vi "FTW-WebServer-Worker-Launch.vi"(0 "Message Handler":refnum<user-event>, 5 "FTW-Endpoint in":refnum<class "FTW-Endpoint.lvclass">, 11 "error in":errorcluster) -> (15 "error out":errorcluster)   [LabVIEW 2015, in "FTW-WebServer.lvclass"]
uses:
  FTW-WebServer.lvclass
  Endpoint/FTW-Endpoint.lvclass
  Message/HttpRequest/FTW-Message-HttpRequest.lvclass
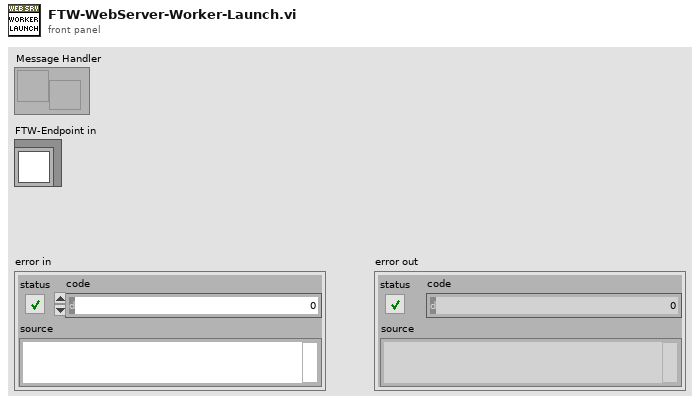
[diagram p1: front panel]
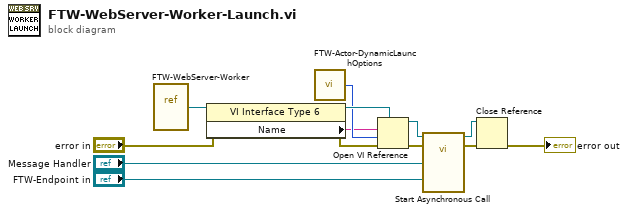
[diagram p0: block diagram]
diagram:
  n1 = vi-ref "FTW-WebServer-Worker.vi"() -> (w1:refnum<vi>)
  n2 = property class="VI Interface Type 6"(reference=w1, error in="error in") -> (reference out=w7:refnum<vi>, error out=w2:errorcluster, "Name"=w3:string)
  n3 = call "FTW-Actor-DynamicLaunchOptions.vi"() -> ("Open VI Ref Options"=w4:i32)
  n4 = Open VI Reference(type specifier VI Refnum (for type only)=w7, vi path=w3, options=w4, error in (no error)=w2) -> (vi reference=w6:refnum<vi>, error out=w5:errorcluster)  [unwired: 2 in]
  n5 = call-by-ref "Start Asynchronous Call"(reference=w6, error in=w5, "Endpoint"="FTW-Endpoint in", "Message Handler"="Message Handler") -> (reference out=w9:refnum<vi>, error out=w8:errorcluster)  [unwired: 1 in]
  n6 = Close Reference(reference=w9, error in (no error)=w8) -> (error out=→"error out":errorcluster)
